vi "Global - UI Stream and Variable Connections.vi"() -> ()   [LabVIEW 2015]
uses:
  Support VIs/Message Queue/Message Cluster.ctl
  Type Definitions/Variable References.ctl
  Support VIs/Message Queue/Message Queue.lvlib
panel:
  in  "Variable References":T1 caption="变量引用"
  in  "UI Stream Reader":refnum<k21> caption="UI网络流读取方端点"
  in  "UI Stream Writer":refnum<k21> caption="UI网络流写入方端点"
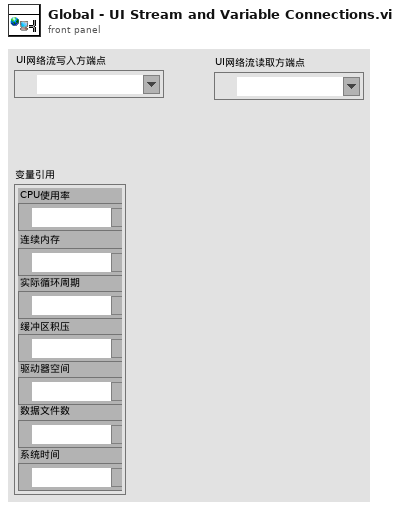
[diagram p1: front panel]
types:
  T1 = typedef "Variable References.ctl" = cluster{"CPU 1 Usage":refnum<k21>, "Free Memory":refnum<k21>, "Actual Loop Period":refnum<k21>, "CPU 2 Usage":refnum<k21>, "Drive Space":refnum<k21>, "Number of Data Files":refnum<k21>, "System Time":refnum<k21>}
diagram:
